vi "Apply Module Limits Pulsed.vi"(8 "error in":errorcluster, 11 "3300 in":refnum<class "3300.lvclass">) -> (0 "error out":errorcluster, 3 "3300 out":refnum<class "3300.lvclass">)   [LabVIEW 2019, in "3300.lvlib" / "3300.lvclass"]
uses:
  Library/3300.lvclass
  C:/Users/Public/Documents/Development/builds/Instruments/Electronic Load.lvlibp/Library/Electronic Load.lvclass
  builds/Instruments/Electronic Load.lvlibp/Private/GUI/Read Trigger_Ref.vi
  Module Support/Access Module Limits.vi
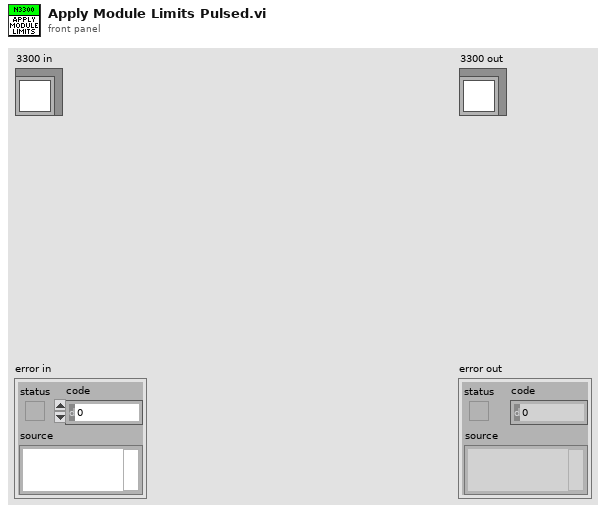
[diagram p1: front panel]
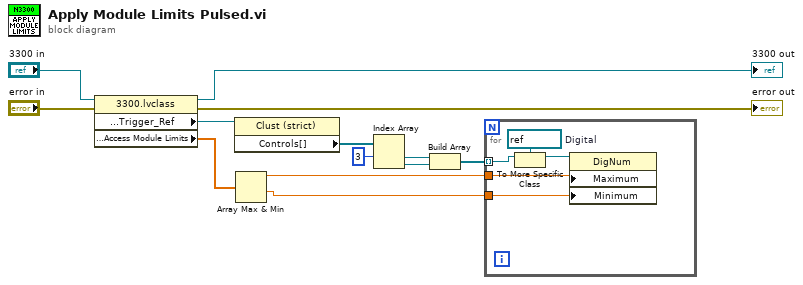
[diagram p0: block diagram]
diagram:
  n1 = property class="3300.lvclass"(reference="3300 in", error in="error in") -> (reference out=→"3300 out":refnum<class "3300.lvclass">, error out=→"error out":errorcluster, "Protected:Accessors:GUI:Trigger_Ref"=w10:refnum<vi>, "Private:Accessors:Access Module Limits"=w11:dbl[])
  n2 = property class="Clust (strict)"(reference=w10) -> ("Controls[]"=w9:refnum<vi>[])  [unwired: 1 in, 2 out]
  n3 = Array Max & Min(array=w11) -> (max value=w7:dbl, min value=w6:dbl)  [unwired: 2 out]
  n4 = Index Array(array=w9, index #1=3 ("index")) -> (element #1=w3:refnum<vi>, element #2=w2:refnum<vi>)  [unwired: 1 in]
  n5 = Build Array(w3, w2) -> (w1:refnum<vi>[])
  n6 = for {
    tunnel: w7 -> [w16]
    tunnel: w6 -> [w15]
    tunnel: w1 -> [w14] mode=indexing
    w17 = refnum<vi> refnum  # Digital
    n7 = To More Specific Class(target class=w17, reference=w14) -> (specific class reference=w18:refnum<vi>)  [unwired: 1 in, 1 out]
    n8 = property class="DigNum"(reference=w18, "Maximum"=w16, "Minimum"=w15) -> ()  [unwired: 1 in, 2 out]
  }
